vi "ep14-events.vi"() -> ()   [LabVIEW 2019]
uses:
  <vilib>/Utility/miscctls.llb/LVPoint32TypeDef.ctl
panel:
  out "ScanCode":i16
  out "Coords":T1
  in  "stop":bool
  out "led":bool
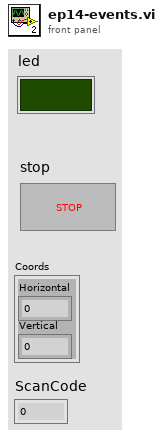
[diagram p1: front panel]
types:
  T1 = typedef "LVPoint32TypeDef.ctl" = cluster{"Horizontal":i32, "Vertical":i32}
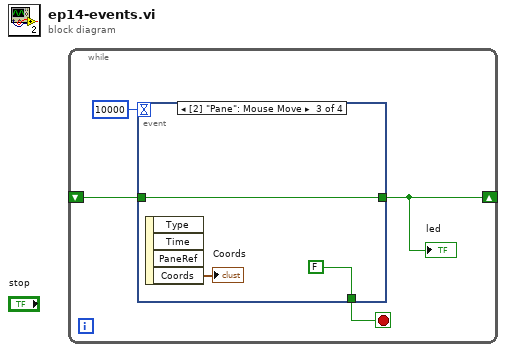
[diagram p0: block diagram]
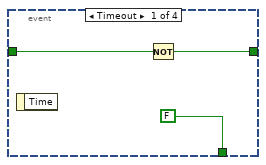
[diagram p2: hidden frame]
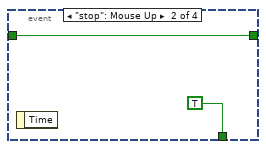
[diagram p3: hidden frame]
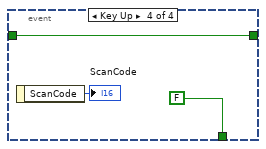
[diagram p4: hidden frame]
diagram:
  n1 = while {
    shift-right: [w2] -> _
    shift-left: _ -> [w3]
    stop <- w1 stop-if-true
    n2 = event shown="[2] \"Pane\": Mouse Move" {
      selector: _ -> [_ _ _ _]
      dyn-events: _ -> [_ _ _ _]
      timeout: 10000 -> [_ _ _ _]
      tunnel: [w7 w8 w11 w14] -> w2
      tunnel: w3 -> [w6 w8 w11 w14]
      tunnel: [FALSE TRUE FALSE FALSE] -> w1
      event Timeout {
        n3 = event-data() -> ()  [unwired: 1 in, 1 out]
        n4 = Not(x=w6) -> (.not. x?=w7:bool)
      }
      event "stop": Mouse Up {
        n5 = event-data() -> ()  [unwired: 1 in, 1 out]
      }
      event Mouse Move {
        n6 = event-data() -> ("Coords"=→"Coords":T1)  [unwired: 1 in, 3 out]
      }
      event Key Up {
        n7 = event-data() -> ("ScanCode"=→"ScanCode":i16)  [unwired: 1 in]
      }
    }
    "led" <- w2
  }
